vi "UVB Serial Read Write.vi"(0 "Transmit":refnum<k21>="Port8/DIO0", 5 "Receive":refnum<k21>="Port8/DIOCTL", 7 "baud rate (115200)":u32=9600, 9 "data bits (8)":i32=8 min=5 max=8 step=1, 12 "stop bits (10: 1 bit)":u16(ring)=10 items=["1.0"=10, "1.5"=15, "2.0"=20], 13 "Invert Polarity?":bool) -> ()   [LabVIEW 2016]
uses:
  <vilib>/rvi/Emulation/niFpgaGetClockAttributes.vi
  <vilib>/rvi/Emulation/niFpgaSctlEmulationGetInTimedLoop.vi
  <vilib>/rvi/Emulation/niFpgaEmulationReportErrorSimple.vi
  <vilib>/rvi/eio/common/nirviEmuTemplateMethod_errors.vi
  <vilib>/rvi/Emulation/niFpgaProcessEmulError.vi
  <vilib>/rvi/Emulation/niFpgaEmulationIsFPGAContextNoSignature.vi
  <vilib>/rvi/errors/niFpgaSetErrorForExecOnDevCompSimple.vi
  <vilib>/rvi/eio/common/nirviEmuReportErrorAndStop.vi
  <vilib>/rvi/DataTransferAndStorage/Container/Common/niFpgaContainerGetUniqueNameForEmu.vi
  <vilib>/rvi/FIFO/Fifo_Resource/nirvififoEmulationSetSize.vi
  <vilib>/rvi/FIFO/Fifo_Resource/nirviFifoEmulationQueueMgr.vi
  <instcachedir>/0/nirviFifoEmulationQueueMgr_E5CAEC123FF24DC58D834DCA3CDAA9B5.lvgen/nirviFifoEmulationQueueMgr_E5CAEC123FF24DC58D834DCA3CDAA9B5_002.vi
  <vilib>/Utility/error.llb/Clear Errors.vi
  <vilib>/rvi/FIFO/Fifo_Resource/nirvififoEmulationCreateLock.vi
  <vilib>/rvi/FIFO/Fifo_Resource/nirvififoEmulationObtainLock.vi
  <vilib>/rvi/FIFO/Fifo_Resource/nirvififoEmulationReleaseLock.vi
  <vilib>/rvi/occurrence/nirviWaitOnOccurrenceBase.vi
  <vilib>/rvi/errors/nirviReportUnexpectedCaseInternalError.vi
  <vilib>/rvi/errors/nirviReportUnexpectedCaseInternalError (U32).vi
  <vilib>/rvi/Emulation/niFpgaCriticalErrorInLSC.vi
  Instance           1 27Saved   LV FPGA Serial Read .vi
  Instance           2 27Saved   LV FPGA Serial Read .vi
  <vilib>/rvi/FIFO/Fifo_Resource/nirvififoEmulationDetermineInputValidOut.vi
  Instance           6 27Saved   LV FPGA Serial Read .vi
  <vilib>/eio/EIOMethodNode/EIOMethodNode.xnode
  <vilib>/rvi/DataTransferAndStorage/Container/XNode/niFpgaContainer.xnode
  <vilib>/rvi/FIFO/Fifo_Resource/nirvififoEmulationRead.vi
  <vilib>/eio/EIONode/EIONode.xnode
  <vilib>/rvi/FIFO/Fifo_Resource/nirvififoEmulationWrite.vi
panel:
  out "Read: Transmission Error":bool
  in  "stop":bool
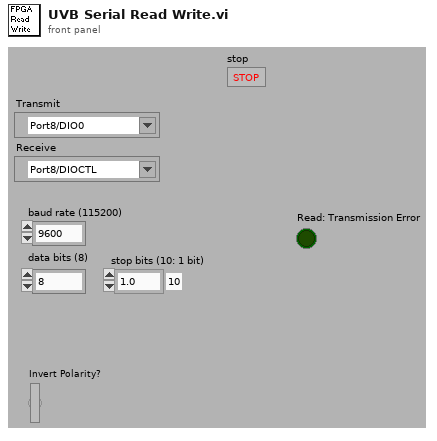
[diagram p1: front panel]
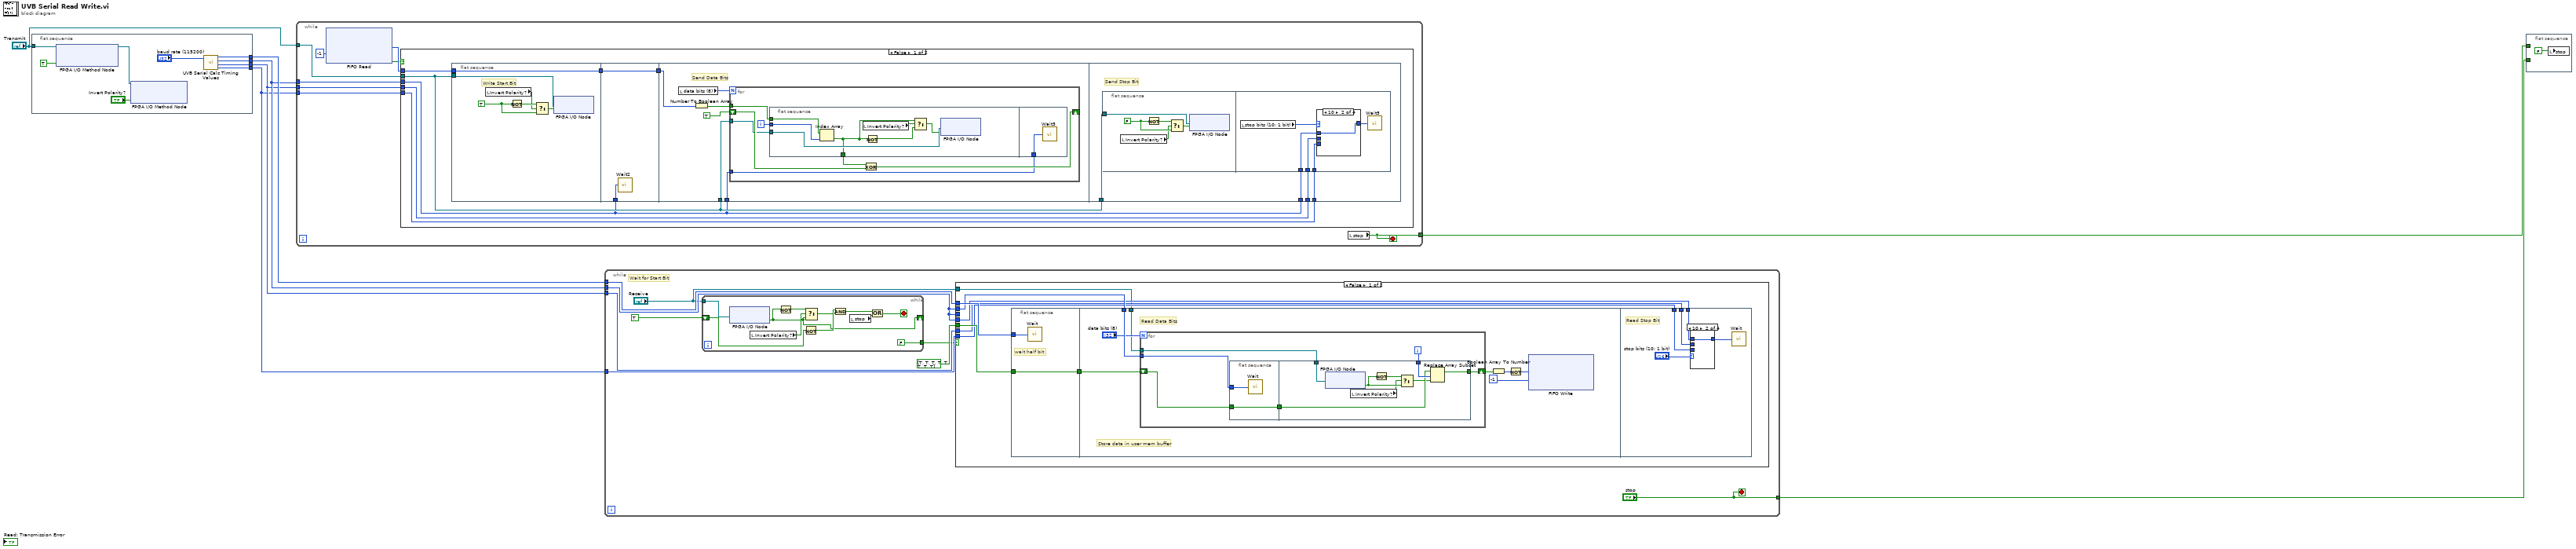
[diagram p0: block diagram]
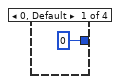
[diagram p2: hidden frame]
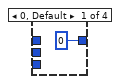
[diagram p6: hidden frame]
diagram:
  n1 = flat-sequence {
    tunnel: [w11] -> w6
    tunnel: [w12] -> w7
    tunnel: [w10] -> w5
    tunnel: [w9] -> w4
    tunnel: "Transmit" -> [w15]
    frame #0 {
      n2 = xnode "FPGA I/O Method Node"("FPGA I/O In"=w15, "Enable"=TRUE ("Digital Enable")) -> ("FPGA I/O Out"=w14:refnum<k21>)
      n3 = xnode "FPGA I/O Method Node"("FPGA I/O In"=w14, "Data"="Invert Polarity?") -> ()  [unwired: 1 out]
      n4 = call "UVB Serial Calc Timing Values.vi"("baud rate (1000000)"="baud rate (115200)") -> ("Two Bit"=w9:u32, "One and Half Bit"=w10:u32, "One Bit"=w11:u32, "Half Bit"=w12:u32)  [unwired: 3 in]
    }
  }
  n5 = while {
    tunnel: w4 -> [w24]
    tunnel: w5 -> [w23]
    tunnel: w6 -> [w22]
    tunnel: "Transmit" -> [w21]
    tunnel: [w18] -> w1
    stop <- w18 stop-if-true
    n6 = xnode ("FIFO Read")("Timeout"=-1) -> ("Element"=w20:u8, "Timed Out?"=w19:bool)  [unwired: 1 in, 1 out]
    n7 = case shown="False" w19 {
      tunnel: w24 -> [w29 _]
      tunnel: w23 -> [w28 _]
      tunnel: w22 -> [w25 _]
      tunnel: w21 -> [w27 _]
      tunnel: w20 -> [w26 _]
      frame False {
        n8 = flat-sequence {
          tunnel: w27 -> [w37]
          tunnel: w26 -> [w32]
          tunnel: [w32] -> w31
          tunnel: w25 -> [w39]
          tunnel: [w38] -> w30
          tunnel: w31 -> [w38]
          tunnel: w30 -> [w40]
          tunnel: w27 -> [w41]
          tunnel: w25 -> [w45]
          tunnel: w25 -> [w64]
          tunnel: w28 -> [w63]
          tunnel: w29 -> [w62]
          tunnel: w27 -> [w61]
          frame #0 {
            w35 = TRUE
            # "Write Start Bit"
            n9 = local read "Invert Polarity?"() -> (w34:bool)
            n10 = Not(x=w35) -> (.not. x?=w36:bool)
            n11 = Select(t=w36, s=w34, f=w35) -> (s? t:f=w33:bool)
            n12 = xnode "FPGA I/O Node"("I/O Item"=w33, "FPGA I/O In"=w37) -> ()  [unwired: 1 out]
          }
          frame #1 {
            n13 = call "Wait2"("Count(Ticks)"=w39) -> ()  [unwired: 1 out]
          }
          frame #2 {
            # "Send Data Bits"
            n14 = local read "data bits (8)"() -> (w42:i32)
            n15 = Number To Boolean Array(number=w40) -> (Boolean array=w43:bool[])
            n16 = for {
              N: w42 -> [_]
              tunnel: w45 -> [w49]
              shift-right: [w52] -> _
              shift-left: TRUE -> [w51]
              tunnel: w43 -> [w48]
              tunnel: w41 -> [w46]
              i -> [w50]
              n17 = flat-sequence {
                tunnel: w50 -> [w59]
                tunnel: w48 -> [w58]
                tunnel: [w53] -> w47
                tunnel: w46 -> [w57]
                tunnel: w49 -> [w60]
                frame #0 {
                  n18 = Index Array(array=w58, index=w59) -> (element=w53:bool)
                  n19 = local read "Invert Polarity?"() -> (w55:bool)
                  n20 = Not(x=w53) -> (.not. x?=w56:bool)
                  n21 = Select(t=w53, s=w55, f=w56) -> (s? t:f=w54:bool)
                  n22 = xnode "FPGA I/O Node"("I/O Item"=w54, "FPGA I/O In"=w57) -> ()  [unwired: 1 out]
                }
                frame #1 {
                  n23 = call "Wait3"("Count(Ticks)"=w60) -> ()  [unwired: 1 out]
                }
              }
              n24 = Exclusive Or(1:w51, 2:w47) -> (0:w52:bool)
            }
          }
          frame #3 {
            # "Send Stop Bit"
            n25 = flat-sequence {
              tunnel: w61 -> [w69]
              tunnel: w62 -> [w72]
              tunnel: w63 -> [w73]
              tunnel: w64 -> [w74]
              frame #0 {
                w67 = FALSE
                n26 = local read "Invert Polarity?"() -> (w66:bool)
                n27 = Not(x=w67) -> (.not. x?=w68:bool)
                n28 = Select(t=w68, s=w66, f=w67) -> (s? t:f=w65:bool)
                n29 = xnode "FPGA I/O Node"("I/O Item"=w65, "FPGA I/O In"=w69) -> ()  [unwired: 1 out]
              }
              frame #1 {
                n30 = local read "stop bits (10: 1 bit)"() -> (w70:u16)
                n31 = case shown="10" w70 {
                  tunnel: w74 -> [_ w76 _ _]
                  tunnel: w73 -> [_ _ w77 _]
                  tunnel: w72 -> [_ _ _ w78]
                  tunnel: [u32 0 ("One Bit") w76 w77 w78] -> w71
                  frame 0, Default {
                  }
                  frame 10 {
                  }
                  frame 15 {
                  }
                  frame 20 {
                  }
                }
                n32 = call "Wait5"("Count(Ticks)"=w71) -> ()  [unwired: 1 out]
              }
            }
          }
        }
      }
      frame True {
      }
    }
    n33 = local read "stop"() -> (w18:bool)
  }
  n34 = while {
    tunnel: w4 -> [w86]
    tunnel: w5 -> [w85]
    tunnel: w6 -> [w84]
    tunnel: w7 -> [w83]
    tunnel: ["stop"] -> w2
    stop <- "stop" stop-if-true
    # "Wait for Start Bit"
    n35 = while {
      tunnel: [FALSE] -> w82
      shift-right: [w88] -> _
      shift-left: TRUE -> [w97]
      tunnel: "Receive" -> [w92]
      stop <- w93 stop-if-true
      n36 = xnode "FPGA I/O Node"("FPGA I/O In"=w92) -> ("I/O Item"=w88:bool)  [unwired: 1 out]
      n37 = local read "Invert Polarity?"() -> (w90:bool)
      n38 = Not(x=w88) -> (.not. x?=w91:bool)
      n39 = Not(x=w97) -> (.not. x?=w96:bool)
      n40 = Select(t=w91, s=w90, f=w88) -> (s? t:f=w89:bool)
      n41 = And(x=w96, y=w89) -> (x .and. y?=w94:bool)
      n42 = local read "stop"() -> (w95:bool)
      n43 = Or(x=w94, y=w95) -> (x .or. y?=w93:bool)
    }
    n44 = case shown="False" w82 {
      tunnel: bool[] [TRUE, TRUE, TRUE, TRUE, TRUE, TRUE, TRUE, TRUE] -> [w106 _]
      tunnel: w83 -> [w105 _]
      tunnel: w84 -> [w104 _]
      tunnel: w84 -> [_ _]
      tunnel: w84 -> [w103 _]
      tunnel: w85 -> [w102 _]
      tunnel: w86 -> [w101 _]
      tunnel: "Receive" -> [w100 _]
      frame False {
        n45 = flat-sequence {
          tunnel: [w108] -> w99
          tunnel: w105 -> [w107]
          tunnel: w106 -> [w108]
          tunnel: w99 -> [w116]
          tunnel: w104 -> [w115]
          tunnel: w100 -> [w111]
          tunnel: w101 -> [w134]
          tunnel: w102 -> [w135]
          tunnel: w103 -> [w136]
          frame #0 {
            # "wait half bit"
            n46 = call "Wait"("Count(Ticks)"=w107) -> ()  [unwired: 1 out]
          }
          frame #1 {
            # "Store data in user mem buffer"
            # "Read Data Bits"
            n47 = for {
              N: "data bits (8)" -> [_]
              shift-right: [w120] -> w114
              shift-left: w116 -> [w122]
              tunnel: w115 -> [w121]
              tunnel: w111 -> [w118]
              i -> [w119]
              n48 = flat-sequence {
                tunnel: w122 -> [w124]
                tunnel: [w124] -> w117
                tunnel: w121 -> [w123]
                tunnel: [w132] -> w120
                tunnel: w118 -> [w128]
                tunnel: w119 -> [w130]
                tunnel: w117 -> [w129]
                frame #0 {
                  n49 = call "Wait"("Count(Ticks)"=w123) -> ()  [unwired: 1 out]
                }
                frame #1 {
                  n50 = xnode "FPGA I/O Node"("FPGA I/O In"=w128) -> ("I/O Item"=w131:bool)  [unwired: 1 out]
                  n51 = local read "Invert Polarity?"() -> (w127:bool)
                  n52 = Not(x=w131) -> (.not. x?=w126:bool)
                  n53 = Select(t=w126, s=w127, f=w131) -> (s? t:f=w125:bool)
                  n54 = Replace Array Subset(array=w129, new element=w125, index=w130) -> (w132:bool[])
                }
              }
            }
            n55 = Boolean Array To Number(Boolean array=w114) -> (number=w113:u8)
            n56 = Not(x=w113) -> (.not. x?=w110:u8)
            n57 = xnode ("FIFO Write")("Element"=w110, "Timeout"=-1) -> ()  [unwired: 1 in, 2 out]
          }
          frame #2 {
            # "Read Stop Bit"
            n58 = case shown="10" "stop bits (10: 1 bit)" {
              tunnel: w136 -> [_ w139 _ _]
              tunnel: w135 -> [_ _ w140 _]
              tunnel: w134 -> [_ _ _ w141]
              tunnel: [u32 0 ("One Bit") w139 w140 w141] -> w133
              frame 0, Default {
              }
              frame 10 {
              }
              frame 15 {
              }
              frame 20 {
              }
            }
            n59 = call "Wait"("Count(Ticks)"=w133) -> ()  [unwired: 1 out]
          }
        }
      }
      frame True {
      }
    }
  }
  n60 = flat-sequence {
    tunnel: w2 -> [_]
    tunnel: w1 -> [_]
    frame #0 {
      n61 = local write "stop"(FALSE ("stop")) -> ()
    }
  }
